vi "Keith 7001 Trig Layer Config.vi"(1 "delay period (sec)":dbl min=0.0 max=99999.999 format="%.3f", 2 "timer interval (sec)":dbl=0.001 min=0.001 max=99999.999 format="%.3f", 3 "trigger link output":u16=2 min=1 max=6 step=1, 4 "trigger link input (/output)":u16=1 min=1 max=6 step=1, 5 "count value":u16=1 min=1 max=9999, 6 "count (auto:0)":u16(ring) items=["auto", "set finite value", "infinite"], 7 "error in":T1, 8 "source bypass":bool, 9 "source (immediate:1)":u16(ring)=1 items=["hold", "immediate", "timer", "manual", "GPIB", "trigger link; asynchronous", "trigger link; semi-synchronous", "external"], 10 "GPIB address":string="7") -> (0 "error out":T1)   [LabVIEW 2019]
doc: "This VI for the Keithley 7001 Switch System sets up the channel layer (trigger layer)."
panel:
  # "enable (source)\ndisable (acceptor)"
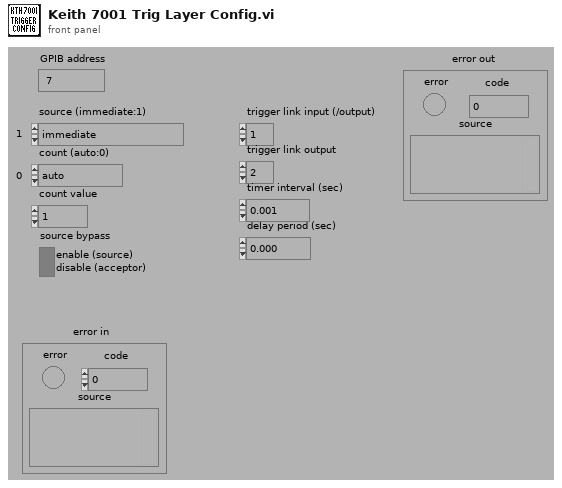
[diagram p1: front panel]
types:
  T1 = cluster{"error":bool, "code":i32, "source":string}
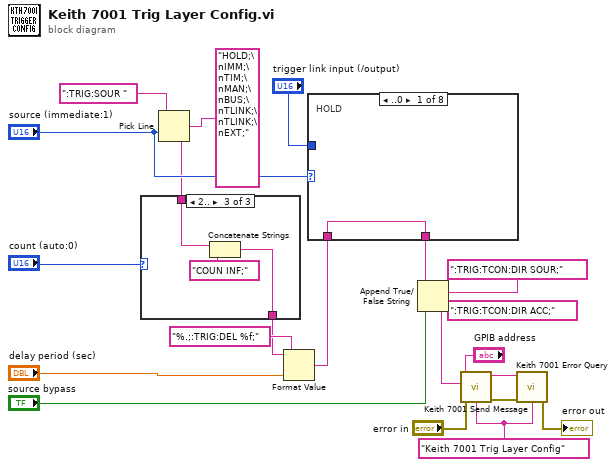
[diagram p0: block diagram]
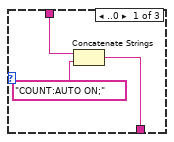
[diagram p2: hidden frame]
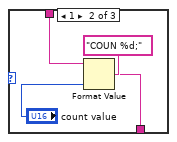
[diagram p3: hidden frame]
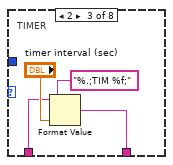
[diagram p5: hidden frame]
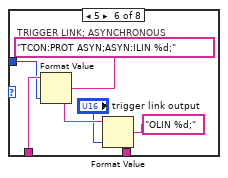
[diagram p8: hidden frame]
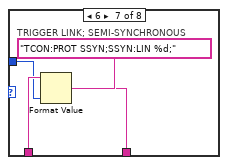
[diagram p9: hidden frame]
diagram:
  w1 = "Keith 7001 Trig Layer Config"
  n1 = Pick Line(string ("")=":TRIG:SOUR ", multi-line string="HOLD;\nIMM;\nTIM;\nMAN;\nBUS;\nTLINK;\nTLINK;\nEXT;", line index="source (immediate:1)") -> (output string=w8:string)
  n2 = case shown="2.." "count (auto:0)" {
    tunnel: w8 -> [w24 w27 w30]
    tunnel: [w22 w25 w29] -> w7
    frame ..0 {
      n3 = Concatenate Strings(w24, "COUNT:AUTO ON;") -> (w22:string)
    }
    frame 1 {
      n4 = Format Value(string ("")=w27, format string="COUN %d;", value (0)="count value") -> (output string=w25:string)
    }
    frame 2.. {
      n5 = Concatenate Strings(w30, "COUN INF;") -> (w29:string)
    }
  }
  n6 = Format Value(string ("")=w7, format string="%.;:TRIG:DEL %f;", value (0)="delay period (sec)") -> (output string=w15:string)
  n7 = case shown="..0" "source (immediate:1)" {
    tunnel: w15 -> [w32 w33 w36 w38 w39 w45 w49 w51]
    tunnel: [w32 w33 w34 w38 w39 w41 w47 w51] -> w13
    tunnel: "trigger link input (/output)" -> [_ _ _ _ _ w40 w48 _]
    frame ..0 {
      # "HOLD"
    }
    frame 1 {
      # "IMMEDIATE"
    }
    frame 2 {
      # "TIMER"
      n8 = Format Value(string ("")=w36, format string="%.;TIM %f;", value (0)="timer interval (sec)") -> (output string=w34:string)
    }
    frame 3 {
      # "MANUAL"
    }
    frame 4 {
      # "GPIB"
    }
    frame 5 {
      # "TRIGGER LINK; ASYNCHRONOUS"
      n9 = Format Value(string ("")=w45, format string="TCON:PROT ASYN;ASYN:ILIN %d;", value (0)=w40) -> (output string=w44:string)
      n10 = Format Value(string ("")=w44, format string="OLIN %d;", value (0)="trigger link output") -> (output string=w41:string)
    }
    frame 6 {
      # "TRIGGER LINK; SEMI-SYNCHRONOUS"
      n11 = Format Value(string ("")=w49, format string="TCON:PROT SSYN;SSYN:LIN %d;", value (0)=w48) -> (output string=w47:string)
    }
    frame 7.. {
      # "EXTERNAL"
    }
  }
  n12 = Append True/False String(1:"source bypass", 2:":TRIG:TCON:DIR ACC;", 3:":TRIG:TCON:DIR SOUR;", 4:w13) -> (0:w10:string)
  n13 = call "Keith 7001 Send Message.vi"("address string"="GPIB address", "write buffer"=w10, "source"=w1, "error in"="error in") -> ("address out"=w4:string, "error out"=w3:T1)  [unwired: 2 in, 2 out]
  n14 = call "Keith 7001 Error Query.vi"("GPIB address"=w4, "error in"=w3, "source"=w1) -> ("error out"=→"error out":T1)  [unwired: 2 out]
